vi "Video Frame Create.vi"(6 "Depth Scale":dbl, 7 "Frame Number":i32, 8 "error in (no error)":errorcluster, 9 "Frame Data":T1, 10 "Image Dst":T2, 11 "Video Frame in":refnum<class "Video Frame.lvclass">) -> (0 "error out":errorcluster, 3 "Video Frame out":refnum<class "Video Frame.lvclass">)   [LabVIEW 2018, in "Video Frame.lvclass"]
uses:
  Video Frame.lvclass
  <vilib>/vision/Image Controls.llb/IMAQ Image.ctl
  Video Frame.lvclass/Video Frame.ctl
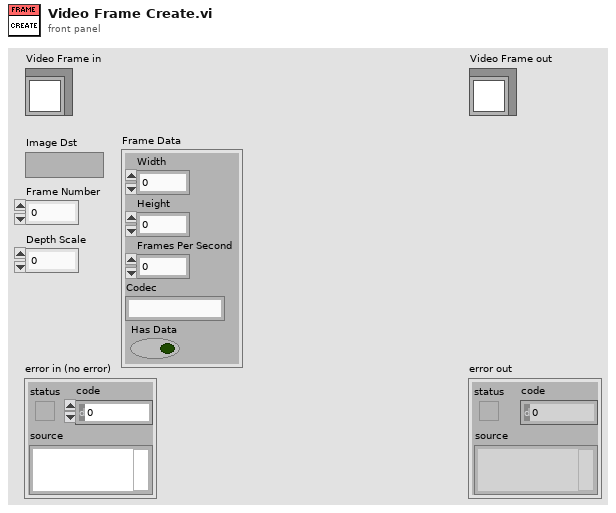
[diagram p1: front panel]
types:
  T1 = cluster{"Width":u32, "Height":u32, "Frames Per Second":u32, "Codec":string, "Has Data":bool}
  T2 = typedef "IMAQ Image.ctl" = refnum<image>
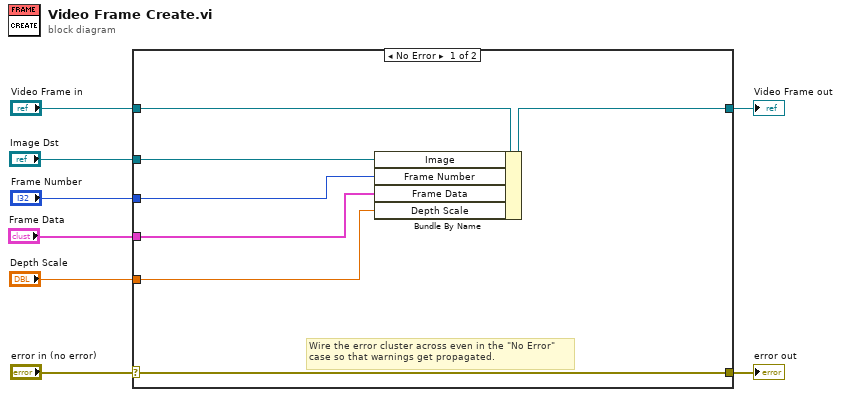
[diagram p0: block diagram]
diagram:
  n1 = case shown="No Error" "error in (no error)" {
    selector: "error in (no error)" -> [w15 w17]
    tunnel: [w15 w17] -> w7
    tunnel: [w9 w16] -> w5
    tunnel: "Video Frame in" -> [w14 w16]
    tunnel: "Image Dst" -> [w13 _]
    tunnel: "Frame Number" -> [w12 _]
    tunnel: "Frame Data" -> [w11 _]
    tunnel: "Depth Scale" -> [w10 _]
    frame No Error {
      # "Wire the error cluster across even in the \"No Error\"\ncase so that warnings get propagated."
      n2 = Bundle By Name(cluster=w14, "Image"=w13, "Frame Number"=w12, "Frame Data"=w11, "Depth Scale"=w10) -> (w9:refnum<class "Video Frame.lvclass">)
    }
    frame Error {
    }
  }
  "error out" <- w7
  "Video Frame out" <- w5
